vi "GFG_Monitor.vi"(8 "error in (no error)":errorcluster) -> (0 "error out":errorcluster)   [LabVIEW 2012, in "GFG library.lvlib"]
uses:
  GFG library.lvlib
panel:
  in  "clear":bool
  in  "Index":dbl
  out "output cluster":cluster{u32[], string[], string[], variant[]}
  in  "Query Variable":string
  in  "Refresh":bool
  out "All Variables":string[](array[string])
  in  "stop":bool
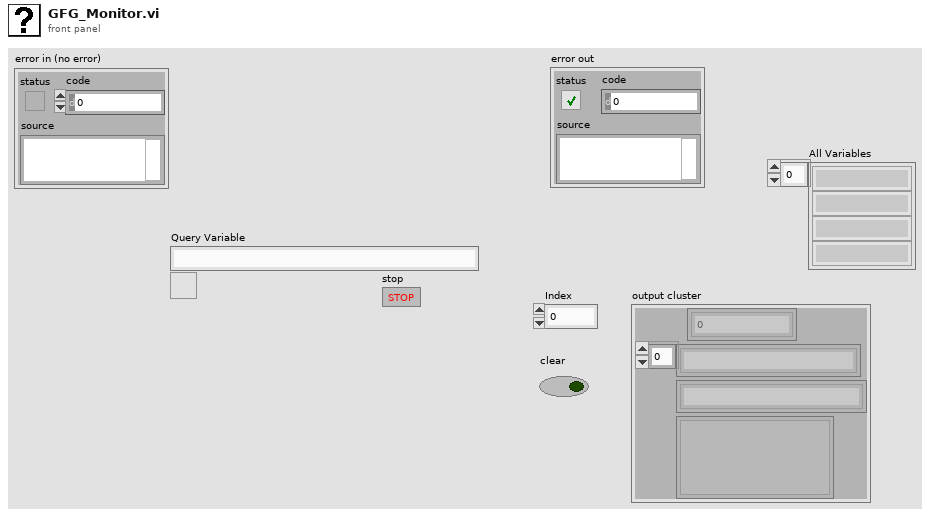
[diagram p1: front panel]
types:
  T1 = typedef "VariantType.lvlib/Type.ctl" = enum8{"Invalid Type", "Void", "I8", "I16", "I32", "I64", "U8", "U16", "U32", "U64", "Single Float", "Double Float", "Extended Float", "Single Complex", "Double Complex", "Extended Complex", "Enum U8", "Enum U16", "Enum U32", "Enum U64", "Single Float With Unit", "Double Float With Unit", "Extended Float With Unit", "Single Complex with Unit", "Double Complex with Unit", "Extended Complex with Unit", "Boolean", "String", "Path", "Picture", "Tag", "Array", "Cluster", "Variant", "LV Variant", "Waveform", "Timestamp", "Digital Waveform", "Digital Data", "ExpressData", "Refnum", "External Data", "VI", "Poly VI", "LabVIEW Class Instance", "Fixed Point"}
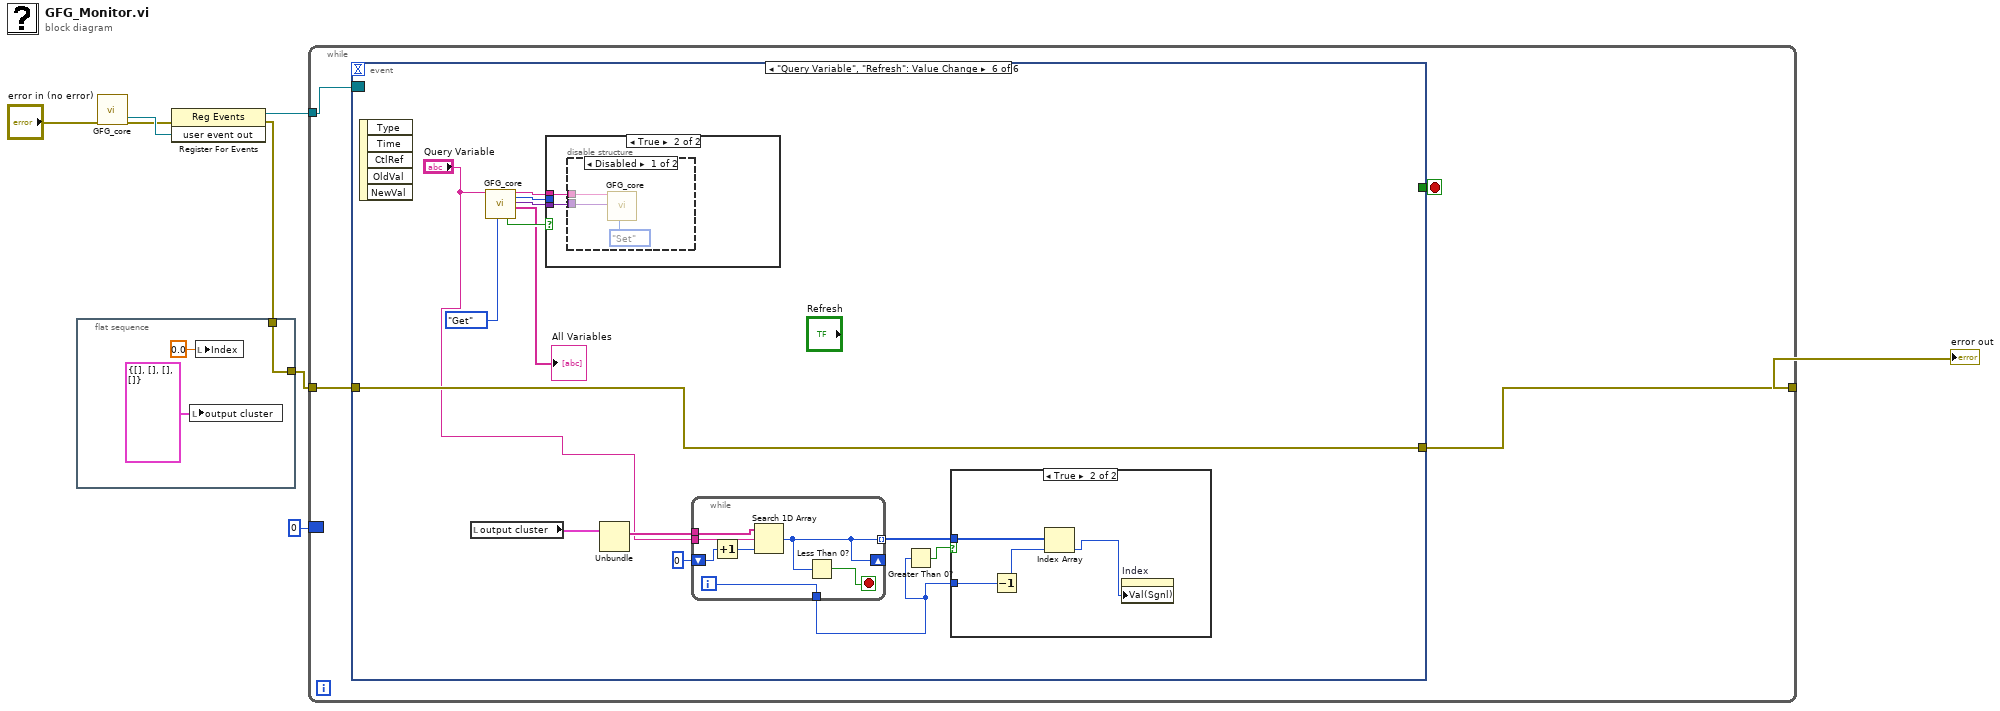
[diagram p0: block diagram]
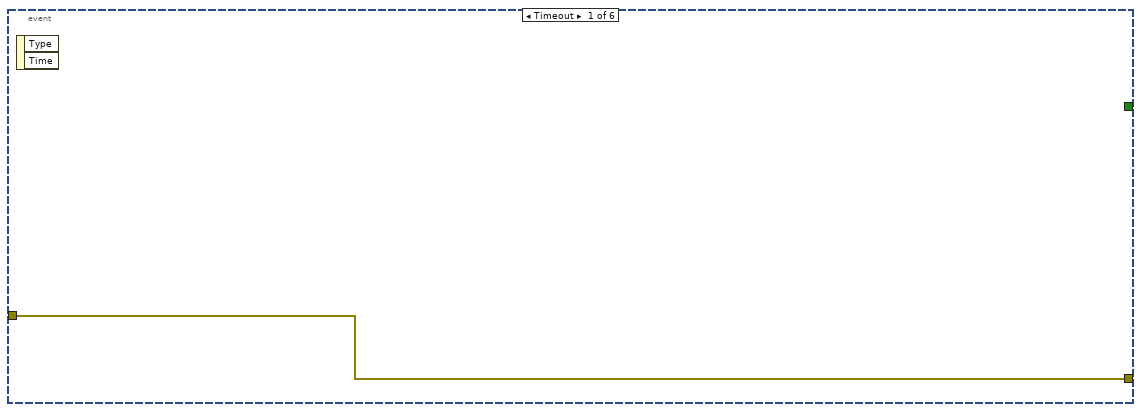
[diagram p2: hidden frame]
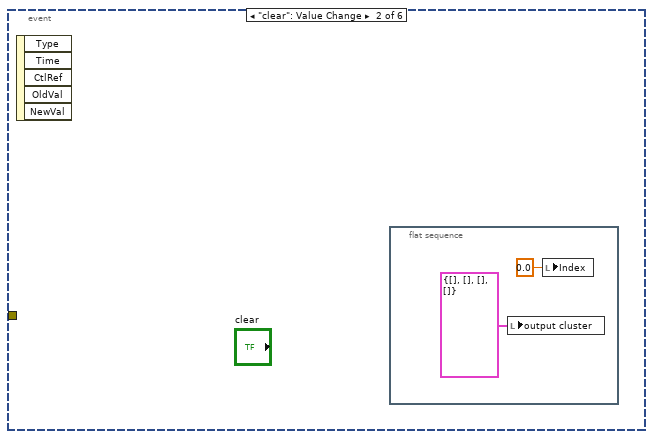
[diagram p3: hidden frame]
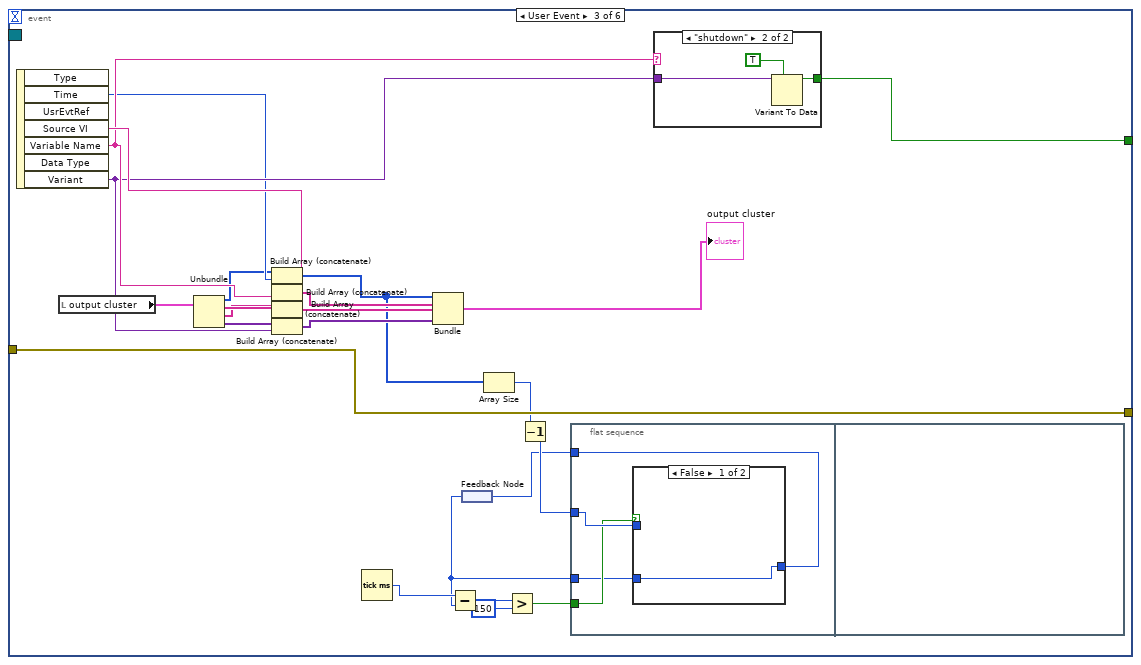
[diagram p4: hidden frame]
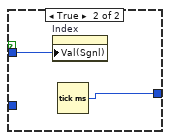
[diagram p5: hidden frame]
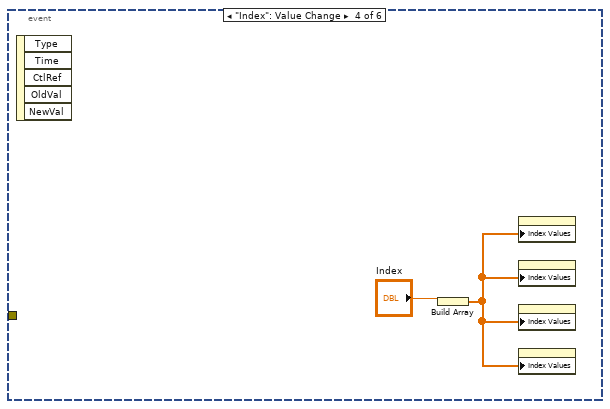
[diagram p7: hidden frame]
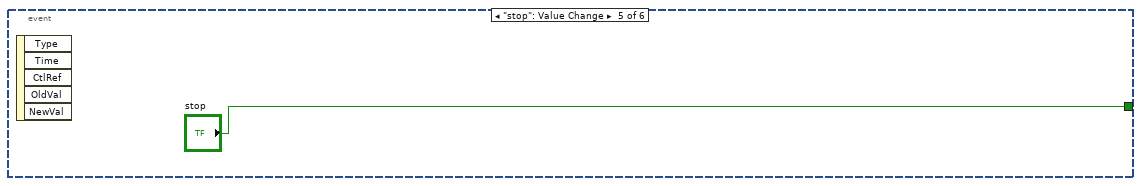
[diagram p8: hidden frame]
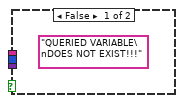
[diagram p10: hidden frame]
diagram:
  n1 = flat-sequence {
    tunnel: [w10] -> w3
    tunnel: w2 -> [w10]
    frame #0 {
      n2 = local write "output cluster"(cluster{u32[], string[], string[], variant[]} {[], [], [], []} ("output cluster")) -> ()
      n3 = local write "Index"(0.0 ("Index")) -> ()
    }
  }
  n4 = call "GFG_core.vi"("error in (no error)"="error in (no error)") -> ("user event out"=w7:refnum<user-event>, "error out"=w6:errorcluster)  [unwired: 12 in, 5 out]
  n5 = register-events(error in=w6, w7) -> (reference out=w8:refnum<event-registration>, error out=w2:errorcluster)  [unwired: 1 in]
  n6 = while {
    tunnel: w8 -> [w15]
    tunnel: w3 -> [w13]
    tunnel: [w12] -> w4
    border: u32 0 ("millisecond timer value") -> [_]
    stop <- w14 stop-if-true
    n7 = event shown="[5] \"Query Variable\", \"Refresh\": Value Change" {
      selector: w15 -> [_ _ _ _ _ _]
      dyn-events: _ -> [_ _ _ _ _ _]
      timeout: _ -> [_ _ _ _ _ _]
      tunnel: [_ _ w42 _ "stop" _] -> w14
      tunnel: w13 -> [w16 _ w41 _ _ w63]
      tunnel: [w16 _ w41 _ _ w63] -> w12
      event Timeout {
        n8 = event-data() -> ()  [unwired: 1 in, 2 out]
      }
      event "clear": Value Change {
        n9 = event-data() -> ()  [unwired: 1 in, 5 out]
        n10 = flat-sequence {
          frame #0 {
            n11 = local write "output cluster"(cluster{u32[], string[], string[], variant[]} {[], [], [], []} ("output cluster")) -> ()
            n12 = local write "Index"(0.0 ("Index")) -> ()
          }
        }
      }
      event User Event {
        n13 = event-data() -> ("Time"=w34:u32, "Source VI"=w40:string, "Variable Name"=w39:string, "Variant"=w38:variant)  [unwired: 1 in, 3 out]
        n14 = local read "output cluster"() -> (w32:cluster{u32[], string[], string[], variant[]})
        n15 = Unbundle(w32) -> (w31:u32[], w30:string[], w29:string[], w28:variant[])
        n16 = Build Array (concatenate)(w31, w34) -> (w27:u32[])
        n17 = Build Array (concatenate)(w30, w39) -> (w37:string[])
        n18 = Build Array (concatenate)(w29, w40) -> (w35:string[])
        n19 = Build Array (concatenate)(w28, w38) -> (w36:variant[])
        n20 = Tick Count (ms)() -> (millisecond timer value=w23:u32)
        n21 = Bundle(w27, w37, w35, w36) -> (→"output cluster":cluster{u32[], string[], string[], variant[]})  [unwired: 1 in]
        n22 = feedback-in #1(w24) -> ()
        n23 = feedback #1() -> (w19:u32)
        n24 = Subtract(x=w23, y=w19) -> (x-y=w22:u32)
        n25 = Array Size(array=w27) -> (size(s)=w26:i32)
        n26 = Greater?(x=w22, y=u32 150) -> (0:w20:bool)
        n27 = Decrement(x=w26) -> (x-1=w25:i32)
        n28 = flat-sequence {
          tunnel: w25 -> [w46]
          tunnel: [w45] -> w24
          tunnel: w20 -> [w44]
          tunnel: w19 -> [w43]
          frame #0 {
            n29 = case shown="False" w44 {
              tunnel: w46 -> [_ w49]
              tunnel: [w47 w48] -> w45
              tunnel: w43 -> [w47 _]
              frame False {
              }
              frame True {
                n30 = property on="Index" class="DigNum (strict)"("Val(Sgnl)"=w49) -> ()  [unwired: 2 in, 2 out]
                n31 = Tick Count (ms)() -> (millisecond timer value=w48:u32)
              }
            }
          }
          frame #1 {
          }
        }
        n32 = case shown="\"shutdown\"" w39 {
          tunnel: w38 -> [_ w52]
          tunnel: [_ w50] -> w42
          frame "False", Default {
          }
          frame "shutdown" {
            n33 = Variant To Data(type=TRUE ("want seconds? (F)"), Variant=w52) -> (data=w50:bool)  [unwired: 1 in, 1 out]
          }
        }
      }
      event "Index": Value Change {
        n34 = event-data() -> ()  [unwired: 1 in, 5 out]
        n35 = Build Array("Index") -> (w53:dbl[])
        n36 = property class="Arr (strict)"("Index Values"=w53) -> ()  [unwired: 2 in, 2 out]
        n37 = property class="Arr (strict)"("Index Values"=w53) -> ()  [unwired: 2 in, 2 out]
        n38 = property class="Arr (strict)"("Index Values"=w53) -> ()  [unwired: 2 in, 2 out]
        n39 = property class="Arr (strict)"("Index Values"=w53) -> ()  [unwired: 2 in, 2 out]
      }
      event "stop": Value Change {
        n40 = event-data() -> ()  [unwired: 1 in, 5 out]
      }
      event "Query Variable", "Refresh": Value Change {
        n41 = event-data() -> ()  [unwired: 1 in, 5 out]
        n42 = local read "output cluster"() -> (w62:cluster{u32[], string[], string[], variant[]})
        n43 = call "GFG_core.vi"("Variable Name in"="Query Variable", "Action"=enum16{"Init", "Set", "Get"}."Get") -> ("Found/Replaced"=w65:bool, "Variable Name Out"=w68:string, "Data Type Out"=w66:T1, "Variant Out"=w67:variant, "All Variable Names Out"=→"All Variables":string[])  [unwired: 11 in, 2 out]
        n44 = case shown="True" w65 {
          tunnel: w68 -> [_ w82]
          tunnel: w67 -> [_ w81]
          tunnel: w66 -> [_ _]
          frame False {
            (unwired) "QUERIED VARIABLE\nDOES NOT EXIST!!!" ("Variable Name Out")
          }
          frame True {
            n45 = disable-structure shown="Disabled" {
              disable-tunnel: w82 -> [w84 _]
              disable-tunnel: w81 -> [w83 _]
              frame Disabled {
                n46 = call "GFG_core.vi"("Variable Name in"=w84, "Variant in"=w83, "Action"=enum16{"Init", "Set", "Get"}."Set") -> ()  [unwired: 10 in, 7 out]
              }
              frame Enabled {
              }
            }
          }
        }
        n47 = Unbundle(w62) -> (w61:string[])  [unwired: 3 out]
        n48 = while {
          tunnel: w61 -> [w80]
          tunnel: "Query Variable" -> [w79]
          tunnel: [w76] -> w59 mode=indexing
          tunnel: [w77] -> w57
          shift-right: [w76] -> _
          shift-left: 0 ("index of element") -> [w75]
          i -> [w77]
          stop <- w78 stop-if-true
          n49 = Increment(x=w75) -> (x+1=w74:i32)
          n50 = Search 1D Array(1D array=w80, element=w79, start index (0)=w74) -> (index of element=w76:i32)
          n51 = Less Than 0?(x=w76) -> (x < 0?=w78:bool)
        }
        n52 = Greater Than 0?(x=w57) -> (x > 0?=w58:bool)
        n53 = case shown="True" w58 {
          tunnel: w59 -> [_ w73]
          tunnel: w57 -> [_ w72]
          frame False {
          }
          frame True {
            n54 = Decrement(x=w72) -> (x-1=w71:i32)
            n55 = Index Array(array=w73, index=w71) -> (element=w70:i32)
            n56 = property on="Index" class="DigNum (strict)"("Val(Sgnl)"=w70) -> ()  [unwired: 2 in, 2 out]
          }
        }
      }
    }
  }
  "error out" <- w4
